vi "ISX3_Example_Configure_Measurementvi.vi"() -> ()   [LabVIEW 2012, in "Sciospec ISX3 Impedance Analyzer.lvlib"]
uses:
  Sciospec ISX3 Impedance Analyzer.lvlib
panel:
  out "ACK for Set Channel":u8[](array[numeric])
  in  "Range Setting":u16(ring)=1 items=["100Ohm"=1, "10kOhm"=2, "1MOhm"=4]
  in  "Measurement Channel":u8(ring)=1 items=["BNC"=1, "ExtensionPort"=2, "ExtensionPort2"=3]
  out "ACK for Save Setup":u8[](array[numeric])
  in  "Save Setup":bool
  in  "Save Slot":u8=1 min=1 step=1
  out "ACK for Add Frequency":u8[](array[numeric])
  out "ACK for Init Setup":u8[](array[numeric])
  in  "Amplitude [V]":sgl=1.0 min=0.001 max=1
  in  "Precision":dbl=1.0 min=0.0
  in  "Frequency Count":sgl=50.0 min=1 max=2048 step=1
  in  "Stop Frequency [Hz]":sgl=1000000.0 min=0.1 max=1e+07
  in  "Start Frequency [Hz]":sgl=100.0 min=0.1 max=1e+07
  in  "Use LogScale":bool=TRUE
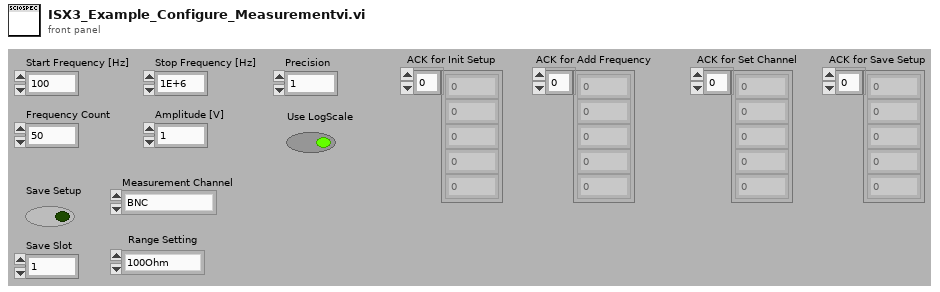
[diagram p1: front panel]
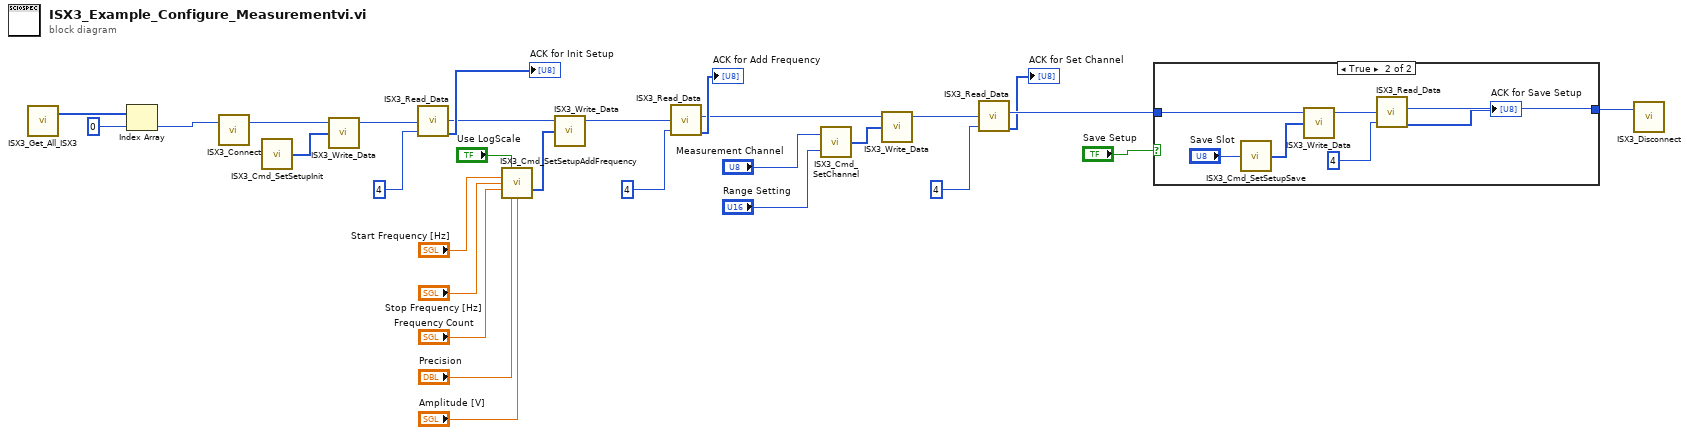
[diagram p0: block diagram]
diagram:
  n1 = call "ISX3_Get_All_ISX3.vi"() -> ("A list of FT_Handel where an ISX-3 is connected to.\nThis handle must be used for further interaction \nwith the USB interface."=w14:u32[])  [unwired: 2 in]
  n2 = Index Array(array=w14, index=u32 0) -> (element=w13:u32)
  n3 = call "ISX3_Connect.vi"("Connect to device with\nFT_Handle"=w13) -> ("Connected to device:"=w12:u32)  [unwired: 2 in]
  n4 = call "ISX3_Cmd_SetSetupInit.vi"() -> ("set Setup Init Cmd"=w10:u8[])  [unwired: 1 in]
  n5 = call "ISX3_Write_Data.vi"("Data to Write"=w10, "FT_Handle"=w12) -> ("FT_Handle"=w11:u32)  [unwired: 2 in, 1 out]
  n6 = call "ISX3_Read_Data.vi"("FT_Handle"=w11, "Bytes To Read"=4) -> ("Handle"=w8:u32, "Read Data"=→"ACK for Init Setup":u8[])  [unwired: 2 in, 1 out]
  n7 = call "ISX3_Cmd_SetSetupAddFrequency.vi"("Use LogScale"="Use LogScale", "Start Frequency [Hz]"="Start Frequency [Hz]", "Stop Frequency [Hz]"="Stop Frequency [Hz]", "Frequency Count"="Frequency Count", "Precision"="Precision", "Amplitude [V]"="Amplitude [V]") -> ("set Setup Init Cmd"=w9:u8[])  [unwired: 9 in]
  n8 = call "ISX3_Write_Data.vi"("Data to Write"=w9, "FT_Handle"=w8) -> ("FT_Handle"=w7:u32)  [unwired: 2 in, 1 out]
  n9 = call "ISX3_Read_Data.vi"("FT_Handle"=w7, "Bytes To Read"=4) -> ("Handle"=w4:u32, "Read Data"=→"ACK for Add Frequency":u8[])  [unwired: 2 in, 1 out]
  n10 = call "ISX3_Cmd_SetChannel.vi"("Range Setting"="Range Setting", "Measurement Channel"="Measurement Channel") -> ("set channel Cmd"=w3:u8[])
  n11 = call "ISX3_Write_Data.vi"("Data to Write"=w3, "FT_Handle"=w4) -> ("FT_Handle"=w2:u32)  [unwired: 2 in, 1 out]
  n12 = call "ISX3_Read_Data.vi"("FT_Handle"=w2, "Bytes To Read"=4) -> ("Handle"=w16:u32, "Read Data"=→"ACK for Set Channel":u8[])  [unwired: 2 in, 1 out]
  n13 = case shown="True" "Save Setup" {
    tunnel: w16 -> [w30 w33]
    tunnel: [w30 w36] -> w1
    frame False {
    }
    frame True {
      n14 = call "ISX3_Cmd_SetSetupSave.vi"("Setup Slot"="Save Slot") -> ("set Setup Save Cmd"=w32:u8[])
      n15 = call "ISX3_Write_Data.vi"("Data to Write"=w32, "FT_Handle"=w33) -> ("FT_Handle"=w31:u32)  [unwired: 2 in, 1 out]
      n16 = call "ISX3_Read_Data.vi"("FT_Handle"=w31, "Bytes To Read"=4) -> ("Handle"=w36:u32, "Read Data"=→"ACK for Save Setup":u8[])  [unwired: 2 in, 1 out]
    }
  }
  n17 = call "ISX3_Disconnect.vi"("FT_Handle"=w1) -> ()  [unwired: 2 in]
